vi "construct_constant_cluster.vi"(1 "Cluster":T1) -> (0 "Limits":T2={"High Charge Limit"=0, "Low Charge Limit"=0, "Time Out Limit"=0, "High Velocity Count"=0, "Low Velocity Count"=0, "Sampling Rate"=26666666.59375, "High Mass Limit"=0, "Low Mass Limit"=0})   [LabVIEW 2015]
uses:
  Limits_In.ctl
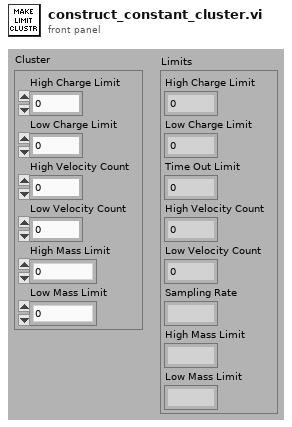
[diagram p1: front panel]
types:
  T1 = typedef "Limits_In.ctl" = cluster{"High Charge Limit":i16, "Low Charge Limit":i16, "High Velocity Count":i32, "Low Velocity Count":i32, "High Mass Limit":i64, "Low Mass Limit":i64}
  T2 = cluster{"High Charge Limit":i16, "Low Charge Limit":i16, "Time Out Limit":u32, "High Velocity Count":i32, "Low Velocity Count":i32, "Sampling Rate":fxp<+,30,25>, "High Mass Limit":i64, "Low Mass Limit":i64}
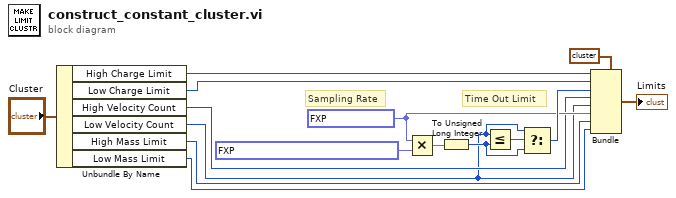
[diagram p0: block diagram]
diagram:
  w10 = fxp<+,30,25> 26666666.59375
  # "Sampling Rate"
  # "Time Out Limit"
  n1 = Unbundle By Name("Cluster") -> ("High Charge Limit"=w6:i16, "Low Charge Limit"=w5:i16, "High Velocity Count"=w4:i32, "Low Velocity Count"=w3:i32, "High Mass Limit"=w2:i64, "Low Mass Limit"=w1:i64)
  n2 = Multiply(x=w10, y=fxp<+,21,-8> 0.0034999996423721313) -> (x*y=w14:fxp<+,51,17>)
  n3 = To Unsigned Long Integer(number=w14) -> (unsigned 32bit integer=w12:u32)
  n4 = Less Or Equal?(x=w3, y=w12) -> (x <= y?=w13:bool)
  n5 = Select(t=w3, s=w13, f=w12) -> (s? t:f=w11:u32)
  n6 = Bundle(cluster=T2 {"High Charge Limit"=0, "Low Charge Limit"=0, "Time Out Limit"=0, "High Velocity Count"=0, "Low Velocity Count"=0, "Sampling Rate"=26666666.59375, "High Mass Limit"=0, "Low Mass Limit"=0} ("Limits"), "High Charge Limit"=w6, "Low Charge Limit"=w5, "Time Out Limit"=w11, "High Velocity Count"=w4, "Low Velocity Count"=w3, "Sampling Rate"=w10, "High Mass Limit"=w2, "Low Mass Limit"=w1) -> (→"Limits":T2)
